vi "例11.6FGEN2.vi"() -> ()   [LabVIEW 2017]
doc: "This example demonstrates how to continuously re-generate analog output data from a buffer in your computer's memory.\n\nRequires Digilent instrumentation product."
uses:
  <vilib>/Utility/error.llb/DialogType.ctl
panel:
  in  "Device Name":string
  in  "Channel":string(combo)="fgen/1"
  in  "Amplitude (V)":dbl=5.0 caption="Amplitude (no change)"
  in  "Frequency (Hz)":dbl=500000.0 caption="Frequency (no change)" format="%#_6p"
  in  "DC Offset (V)":dbl caption="DC Offset (no change)"
  # "MSO Channel Settings"
  # "Sine Wave Sweep Settings"
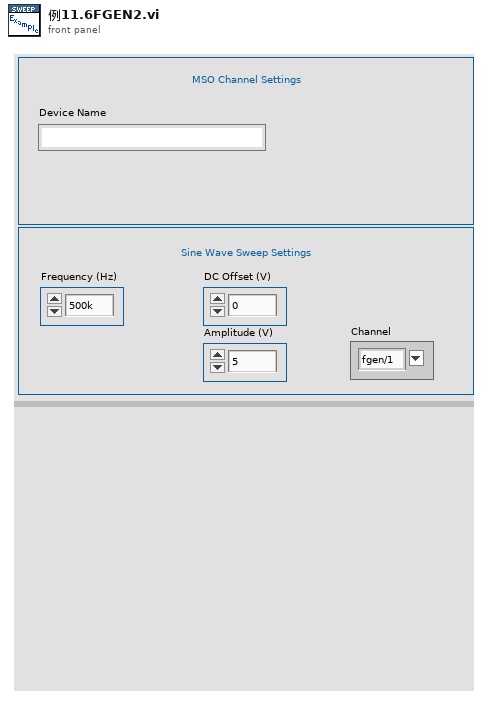
[diagram p1: front panel]
types:
  T1 = typedef "DialogType.ctl" = u16
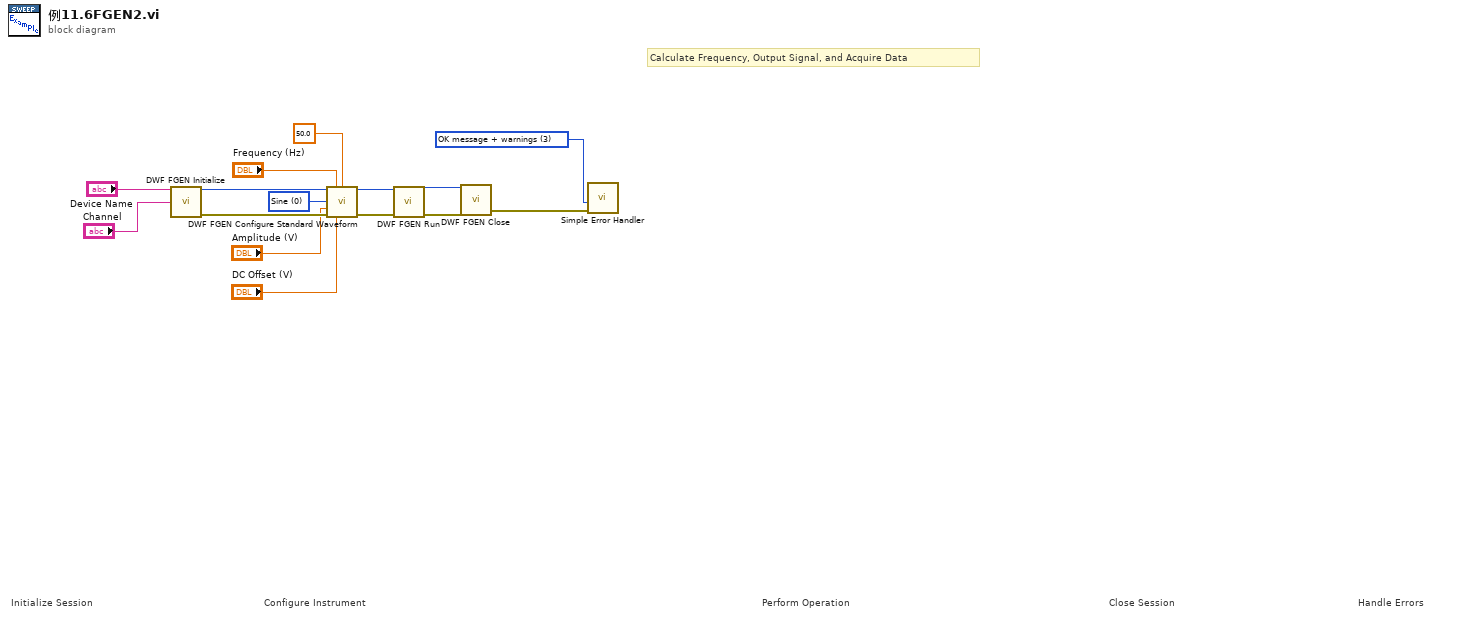
[diagram p0: block diagram]
diagram:
  w6 = 0 items=["Sine", "Square", "Triangle/Ramp", "DC"] ("Waveform Function")
  w15 = T1 3 items=["no dialog", "OK message", "continue or stop message", "OK message + warnings", "continue/stop + warnings"] ("type of dialog (OK msg:1)")
  # "Calculate Frequency, Output Signal, and Acquire Data"
  # "Handle Errors"
  # "Close Session"
  # "Perform Operation"
  # "Configure Instrument"
  # "Initialize Session"
  n1 = call <vilib>:"DWF FGEN Initialize.vi"("Device Name"="Device Name", "Channel"="Channel") -> ("Instrument Handle Out"=w13:u32, "Error Out"=w14:errorcluster)  [unwired: 12 in]
  n2 = call <vilib>:"DWF FGEN Configure Standard Waveform.vi"("Instrument Handle In"=w13, "Frequency"="Frequency (Hz)", "Duty Cycle"=50.0, "Waveform Function"=w6, "Amplitude"="Amplitude (V)", "Error In"=w14, "DC Offset"="DC Offset (V)") -> ("Instrument Handle Out"=w11:u32, "Error Out"=w10:errorcluster)  [unwired: 7 in]
  n3 = call <vilib>:"DWF FGEN Run.vi"("Instrument Handle In"=w11, "Error In"=w10) -> ("Instrument Handle Out"=w2:u32, "Error Out"=w1:errorcluster)  [unwired: 12 in]
  n4 = call <vilib>:"DWF FGEN Close.vi"("Instrument Handle In"=w2, "Error In"=w1) -> ("Error Out"=w3:errorcluster)  [unwired: 13 in]
  n5 = call <vilib>:"Simple Error Handler.vi"("type of dialog (OK msg:1)"=w15, "error in (no error)"=w3) -> ()  [unwired: 3 in, 5 out]
